vi "Check State.vi"(8 "error in (no error)":errorcluster, 11 "Timed Data in":refnum<class "Timed Data.lvclass">) -> (0 "error out":errorcluster, 2 "Previously Populated?":bool, 3 "Timed Data out":refnum<class "Timed Data.lvclass">)   [LabVIEW 2020, in "Publisher.lvlib" / "Timed Data.lvclass"]
doc: "Check if the Timed data has been populated already.\nA Data ID greater than 0 will return Previously Populated? = TRUE."
uses:
  Timed Data.lvclass
  Timed Data.lvclass/Timed Data.ctl
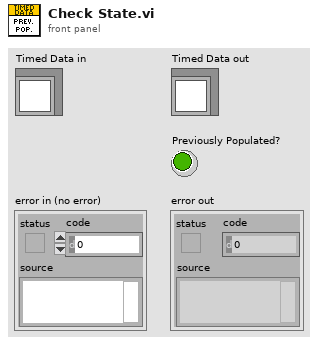
[diagram p1: front panel]
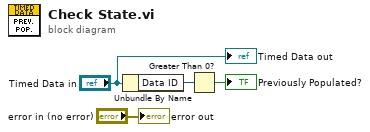
[diagram p0: block diagram]
diagram:
  n1 = Unbundle By Name("Timed Data in") -> ("Data ID"=w2:u32)
  n2 = Greater Than 0?(x=w2) -> (x > 0?=→"Previously Populated?":bool)
  "error out" <- "error in (no error)"
  "Timed Data out" <- "Timed Data in"
